vi "DataTreeCtrl loadedDoc.vi"(8 "error in (no error)":errorcluster, 10 "RootPath":path, 11 "DataTreeCtrl in":refnum<class "DataTreeCtrl.lvclass">) -> (0 "error out":errorcluster, 3 "DataTreeCtrl out":refnum<class "DataTreeCtrl.lvclass">)   [LabVIEW 2018, in "DataTreeCtrl.lvclass"]
uses:
  DataTreeCtrl.lvclass
  <vilib>/picture/picture.llb/imagedata.ctl
  DataTreeCtrl.lvclass/DataTreeCtrl.ctl
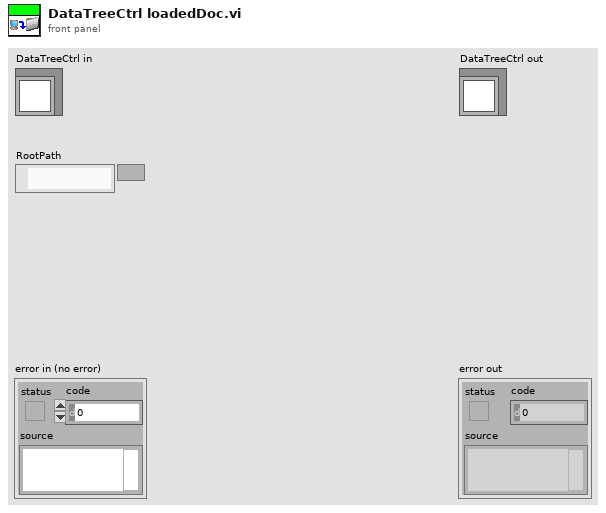
[diagram p1: front panel]
types:
  T1 = cluster{"Left Cell String":string, "Child Text":string[], "Child Tag":string, "Item Indent":i32, "Child Only?":bool, "Glyph Index":i32}
  T2 = typedef "imagedata.ctl" = cluster{"image type":i32, "image depth":i32, "image":u8[], "mask":u8[], "colors":u32[], "Rectangle":cluster{"left":i16, "top":i16, "right":i16, "bottom":i16}}
  T3 = cluster{"Left Cell String":string, "Child Text":string[], "Child Tag":string, "Item Indent":i32, "Child Only?":bool, "Glyph Index":i32}[]
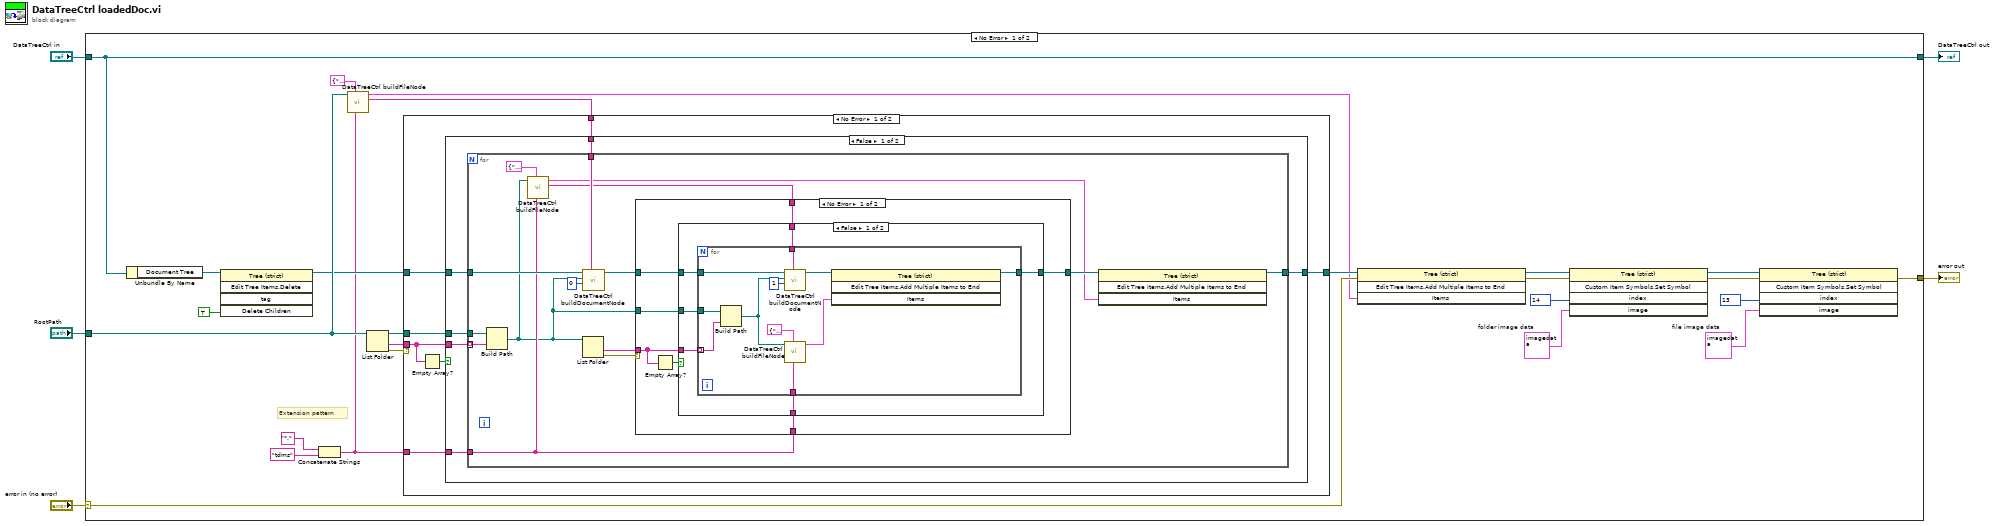
[diagram p0: block diagram]
diagram:
  n1 = case shown="No Error" "error in (no error)" {
    selector: "error in (no error)" -> [w19 w88]
    tunnel: [w17 w88] -> w1
    tunnel: [w10 w87] -> w4
    tunnel: "DataTreeCtrl in" -> [w10 w87]
    tunnel: "RootPath" -> [w13 _]
    frame No Error {
      w28 = T2 {"image type"=0, "image depth"=32, "image"=[0, 0, 0, 0, 0, 0, 0, 0, 0, 0, 0, 0, 0, 0, 0, 0, 0, 0, 0, 0, 0, 0, 0, 0, 0, 0, 0, 0, 0, 0, 0, 0, 0, 0, 0, 0, 0, 0, 0, 0, 0, 0, 0, 0, 0, 0, 0, 0, 0, 0, 0, 0, 0, 0, 0, 0, 0, 0, 0, 0, 0, 0, 0, 0, 0, 0, 0, 0, 0, 0, 0, 0, 0, 0, 0, 0, 0, 0, 0, 0, 0, 0, 0, 0, 0, 0, 0, 0, 0, 0, 0, 0, 0, 0, 0, 0, 0, 0, 0, 0, 0, 0, 0, 0, 0, 0, 0, 0, 0, 0, 0, 0, 0, 0, 0, 0, 0, 0, 0, 0, 0, 0, 0, 0, 0, 0, 0, 0, 0, 0, 0, 0, 0, 0, 0, 0, 0, 0, 0, 0, 0, 0, 0, 0, 0, 0, 0, 0, 0, 0, 0, 0, 0, 0, 0, 0, 0, 0, 0, 0, 0, 0, 0, 0, 0, 0, 0, 0, 0, 0, 0, 0, 0, 0, 0, 0, 0, 0, 0, 0, 0, 0, 0, 0, 0, 0, 0, 0, 0, 0, 0, 0, 0, 0, 0, 0, 0, 0, 0, 0, 0, 0, 0, 0, 0, 0, 0, 0, 0, 0, 0, 0, 0, 0, 0, 0, 0, 0, 0, 0, 0, 0, 0, 0, 0, 0, 0, 0, 0, 0, 0, 0, 0, 0, 0, 0, 255, 0, 141, 202, 0, 0, 0, 0, 0, 0, 0, 0, 0, 0, 0, 0, 0, 0, 0, 0, 0, 0, 0, 0, 0, 0, 0, 0, 0, 0, 0, 0, 0, 0, 0, 0, 0, 0, 0, 0, 0, 0, 0, 0, 0, 0, 0, 0, 0, 0, 0, 0, 0, 0, 0, 0, 0, 0, 0, 0, 0, 0, 0, 0, 255, 0, 141, 202, 0, 0, 0, 0, 0, 0, 0, 0, 0, 0, 0, 0, 0, 0, 0, 0, 0, 0, 0, 0, 0, 0, 0, 0, 0, 0, 0, 0, 0, 0, 0, 0, 0, 0, 0, 0, 0, 0, 0, 0, 0, 0, 0, 0, 0, 0, 0, 0, 0, 0, 0, 0, 0, 0, 0, 0, 0, 0, 0, 0, 255, 0, 141, 202, 0, 0, 0, 0, 0, 0, 0, 0, 0, 0, 0, 0, 0, 0, 0, 0, 0, 0, 0, 0, 0, 0, 0, 0, 0, 0, 0, 0, 0, 0, 0, 0, 0, 0, 0, 0, 0, 0, 0, 0, 0, 0, 0, 0, 0, 0, 0, 0, 0, 0, 0, 0, 0, 0, 0, 0, 0, 0, 0, 0, 255, 0, 141, 202, 0, 0, 0, 0, 0, 0, 0, 0, 0, 0, 0, 0, 0, 0, 0, 0, 0, 0, 0, 0, 0, 0, 0, 0, 0, 0, 0, 0, 0, 0, 0, 0, 0, 0, 0, 0, 0, 0, 0, 0, 0, 0, 0, 0, 255, 0, 141, 202, 0, 0, 0, 0, 0, 0, 0, 0, 0, 0, 0, 0, 255, 0, 141, 202, 0, 0, 0, 0, 0, 0, 0, 0, 0, 0, 0, 0, 255, 0, 141, 202, 0, 0, 0, 0, 0, 0, 0, 0, 0, 0, 0, 0, 0, 0, 0, 0, 0, 0, 0, 0, 0, 0, 0, 0, 0, 0, 0, 0, 255, 0, 141, 202, 0, 0, 0, 0, 0, 0, 0, 0, 0, 0, 0, 0, 255, 0, 141, 202, 0, 0, 0, 0, 255, 0, 141, 202, 0, 0, 0, 0, 255, 0, 141, 202, 0, 0, 0, 0, 0, 0, 0, 0, 0, 0, 0, 0, 0, 0, 0, 0, 0, 0, 0, 0, 0, 0, 0, 0, 0, 0, 0, 0, 255, 0, 141, 202, 0, 0, 0, 0, 0, 0, 0, 0, 0, 0, 0, 0, 255, 0, 141, 202, 0, 0, 0, 0, 255, 0, 141, 202, 0, 0, 0, 0, 255, 0, 141, 202, 0, 0, 0, 0, 0, 0, 0, 0, 0, 0, 0, 0, 255, 0, 141, 202, 0, 0, 0, 0, 0, 0, 0, 0, 0, 0, 0, 0, 255, 0, 141, 202, 0, 0, 0, 0, 0, 0, 0, 0, 0, 0, 0, 0, 255, 0, 141, 202, 0, 0, 0, 0, 255, 0, 141, 202, 0, 0, 0, 0, 255, 0, 141, 202, 0, 0, 0, 0, 255, 0, 141, 202, 0, 0, 0, 0, 255, 0, 141, 202, 0, 0, 0, 0, 0, 0, 0, 0, 0, 0, 0, 0, 255, 0, 141, 202, 0, 0, 0, 0, 255, 0, 141, 202, 0, 0, 0, 0, 255, 0, 141, 202, 0, 0, 0, 0, 255, 0, 141, 202, 0, 0, 0, 0, 255, 0, 141, 202, 0, 0, 0, 0, 255, 0, 141, 202, 0, 0, 0, 0, 255, 0, 141, 202, 0, 0, 0, 0, 255, 0, 141, 202, 0, 0, 0, 0, 255, 0, 141, 202, 0, 0, 0, 0, 255, 0, 141, 202, 0, 0, 0, 0, 255, 0, 141, 202, 0, 0, 0, 0, 255, 0, 141, 202, 0, 0, 0, 0, 255, 0, 141, 202, 0, 0, 0, 0, 255, 0, 141, 202, 0, 0, 0, 0, 255, 0, 141, 202, 0, 0, 0, 0, 255, 0, 141, 202, 0, 0, 0, 0, 255, 0, 141, 202, 0, 0, 0, 0, 255, 0, 141, 202, 0, 0, 0, 0, 255, 0, 141, 202, 0, 0, 0, 0, 255, 0, 141, 202, 0, 0, 0, 0, 255, 0, 141, 202, 255, 0, 0, 0, 255, 0, 0, 0, 255, 0, 0, 0, 255, 0, 0, 0, 255, 0, 0, 0, 255, 0, 0, 0, 255, 0, 0, 0, 255, 0, 0, 0, 255, 0, 0, 0, 255, 0, 0, 0, 255, 0, 0, 0, 255, 0, 0, 0, 255, 0, 0, 0, 255, 0, 0, 0, 255, 0, 0, 0, 255, 0, 0, 0, 0, 0, 0, 0, 0, 0, 0, 0, 0, 0, 0, 0, 0, 0, 0, 0, 0, 0, 0, 0, 0, 0, 0, 0, 0, 0, 0, 0, 0, 0, 0, 0, 0, 0, 0, 0, 0, 0, 0, 0, 0, 0, 0, 0, 0, 0, 0, 0, 0, 0, 0, 0, 0, 0, 0, 0, 0, 0, 0, 0, 0, 0, 0, 0], "mask"=[0, 0, 0, 0, 0, 0, 0, 16, 0, 16, 0, 16, 0, 16, 1, 17, 1, 21, 1, 21, 17, 21, 81, 85, 85, 85, 85, 85, 255, 255, 0, 0], "colors"=[], "Rectangle"={"left"=0, "top"=0, "right"=16, "bottom"=16}}  # file image data
      w27 = T2 {"image type"=0, "image depth"=32, "image"=[16, 0, 0, 0, 16, 0, 0, 0, 16, 0, 0, 0, 16, 0, 0, 0, 16, 0, 0, 0, 12, 0, 0, 0, 0, 0, 0, 0, 0, 0, 0, 0, 0, 0, 0, 0, 0, 0, 0, 0, 0, 0, 0, 0, 0, 0, 0, 0, 0, 0, 0, 0, 0, 0, 0, 0, 0, 0, 0, 0, 0, 0, 0, 0, 255, 0, 0, 0, 255, 0, 0, 0, 255, 0, 0, 0, 255, 0, 0, 0, 255, 0, 0, 0, 248, 0, 0, 0, 44, 0, 0, 0, 0, 0, 0, 0, 0, 0, 0, 0, 0, 0, 0, 0, 0, 0, 0, 0, 0, 0, 0, 0, 0, 0, 0, 0, 0, 0, 0, 0, 0, 0, 0, 0, 0, 0, 0, 0, 255, 0, 0, 0, 255, 0, 0, 0, 255, 0, 0, 0, 255, 0, 0, 0, 255, 0, 0, 0, 255, 0, 0, 0, 209, 0, 0, 0, 48, 0, 0, 0, 48, 0, 0, 0, 48, 0, 0, 0, 48, 0, 0, 0, 48, 0, 0, 0, 48, 0, 0, 0, 48, 0, 0, 0, 48, 0, 0, 0, 48, 0, 0, 0, 255, 0, 0, 0, 255, 0, 0, 0, 255, 0, 0, 0, 255, 0, 0, 0, 255, 0, 0, 0, 255, 0, 0, 0, 255, 0, 0, 0, 202, 0, 0, 0, 88, 0, 0, 0, 88, 0, 0, 0, 88, 0, 0, 0, 88, 0, 0, 0, 88, 0, 0, 0, 88, 0, 0, 0, 88, 0, 0, 0, 177, 0, 0, 0, 255, 0, 0, 0, 255, 0, 0, 0, 255, 0, 0, 0, 255, 0, 0, 0, 255, 0, 0, 0, 255, 0, 0, 0, 255, 0, 0, 0, 254, 0, 0, 0, 116, 0, 0, 0, 88, 0, 0, 0, 88, 0, 0, 0, 88, 0, 0, 0, 88, 0, 0, 0, 88, 0, 0, 0, 88, 0, 0, 0, 177, 0, 0, 0, 255, 0, 0, 0, 255, 0, 0, 0, 255, 0, 0, 0, 255, 0, 0, 0, 255, 0, 0, 0, 255, 0, 0, 0, 255, 0, 0, 0, 255, 0, 0, 0, 255, 0, 0, 0, 255, 0, 0, 0, 255, 0, 0, 0, 255, 0, 0, 0, 255, 0, 0, 0, 255, 0, 0, 0, 255, 0, 0, 0, 255, 0, 0, 0, 255, 0, 0, 0, 255, 0, 0, 0, 255, 0, 0, 0, 255, 0, 0, 0, 255, 0, 0, 0, 255, 0, 0, 0, 255, 0, 0, 0, 255, 0, 0, 0, 255, 0, 0, 0, 255, 0, 0, 0, 255, 0, 0, 0, 255, 0, 0, 0, 255, 0, 0, 0, 255, 0, 0, 0, 255, 0, 0, 0, 255, 0, 0, 0, 255, 0, 0, 0, 255, 0, 0, 0, 255, 0, 0, 0, 255, 0, 0, 0, 246, 0, 0, 0, 152, 0, 0, 0, 152, 0, 0, 0, 152, 0, 0, 0, 157, 0, 0, 0, 254, 0, 0, 0, 255, 0, 0, 0, 255, 0, 0, 0, 255, 0, 0, 0, 255, 0, 0, 0, 255, 0, 0, 0, 255, 0, 0, 0, 255, 0, 0, 0, 255, 0, 0, 0, 255, 0, 0, 0, 255, 0, 0, 0, 255, 0, 0, 0, 224, 0, 0, 0, 224, 0, 0, 0, 224, 0, 0, 0, 228, 0, 0, 0, 255, 0, 0, 0, 255, 0, 0, 0, 255, 0, 0, 0, 255, 0, 0, 0, 255, 0, 0, 0, 255, 0, 0, 0, 255, 0, 0, 0, 255, 0, 0, 0, 255, 0, 0, 0, 255, 0, 0, 0, 255, 0, 0, 0, 246, 0, 0, 0, 121, 0, 0, 0, 120, 0, 0, 0, 120, 0, 0, 0, 120, 0, 0, 0, 120, 0, 0, 0, 121, 0, 0, 0, 246, 0, 0, 0, 255, 0, 0, 0, 255, 0, 0, 0, 255, 0, 0, 0, 255, 0, 0, 0, 255, 0, 0, 0, 255, 0, 0, 0, 255, 0, 0, 0, 255, 0, 0, 0, 254, 0, 0, 0, 208, 0, 0, 0, 208, 0, 0, 0, 208, 0, 0, 0, 208, 0, 0, 0, 208, 0, 0, 0, 208, 0, 0, 0, 254, 0, 0, 0, 255, 0, 0, 0, 255, 0, 0, 0, 255, 0, 0, 0, 255, 0, 0, 0, 255, 0, 0, 0, 255, 0, 0, 0, 255, 0, 0, 0, 255, 0, 0, 0, 248, 0, 0, 0, 168, 0, 0, 0, 168, 0, 0, 0, 168, 0, 0, 0, 168, 0, 0, 0, 168, 0, 0, 0, 168, 0, 0, 0, 248, 0, 0, 0, 255, 0, 0, 0, 255, 0, 0, 0, 255, 0, 0, 0, 255, 0, 0, 0, 255, 0, 0, 0, 255, 0, 0, 0, 255, 0, 0, 0, 255, 0, 0, 0, 255, 0, 0, 0, 255, 0, 0, 0, 255, 0, 0, 0, 255, 0, 0, 0, 255, 0, 0, 0, 255, 0, 0, 0, 255, 0, 0, 0, 255, 0, 0, 0, 255, 0, 0, 0, 255, 0, 0, 0, 255, 0, 0, 0, 255, 0, 0, 0, 255, 0, 0, 0, 255, 0, 0, 0, 255, 0, 0, 0, 255, 0, 0, 0, 255, 0, 0, 0, 255, 0, 0, 0, 255, 0, 0, 0, 255, 0, 0, 0, 255, 0, 0, 0, 255, 0, 0, 0, 255, 0, 0, 0, 255, 0, 0, 0, 255, 0, 0, 0, 255, 0, 0, 0, 255, 0, 0, 0, 255, 0, 0, 0, 255, 0, 0, 0, 255, 0, 0, 0, 255, 0, 0, 0, 255, 0, 0, 0, 255, 0, 0, 0, 255, 0, 0, 0, 255, 0, 0, 0, 255, 0, 0, 0, 255, 0, 0, 0, 255, 0, 0, 0, 255, 0, 0, 0, 255, 0, 0, 0, 255, 0, 0, 0, 255, 0, 0, 0, 255, 0, 0, 0, 255, 0, 0, 0, 16, 0, 0, 0, 16, 0, 0, 0, 16, 0, 0, 0, 16, 0, 0, 0, 16, 0, 0, 0, 16, 0, 0, 0, 16, 0, 0, 0, 16, 0, 0, 0, 16, 0, 0, 0, 16, 0, 0, 0, 16, 0, 0, 0, 16, 0, 0, 0, 16, 0, 0, 0, 16, 0, 0, 0, 16, 0, 0, 0, 16, 0, 0, 0], "mask"=[0, 0, 252, 0, 254, 0, 255, 1, 255, 1, 255, 255, 255, 255, 255, 255, 255, 255, 248, 31, 255, 255, 255, 255, 255, 255, 255, 255, 255, 255, 0, 0], "colors"=[], "Rectangle"={"left"=0, "top"=0, "right"=16, "bottom"=16}}  # folder image data
      # "Extension pattern"
      n2 = Unbundle By Name(w10) -> ("Document Tree"=w12:refnum<vi>)
      n3 = invoke class="Tree (strict)" method="Edit Tree Items.Delete"(reference=w12, "Delete Children"=TRUE ("Delete Children?")) -> (reference out=w9:refnum<vi>)  [unwired: 3 in, 4 out]
      n4 = Concatenate Strings("*." ("string"), "tdms" ("string")) -> (w6:string)
      n5 = call "DataTreeCtrl buildFileNode.vi"("Extension pattern"=w6, "Item"=T1 {"Left Cell String"="", "Child Text"=[], "Child Tag"="", "Item Indent"=0, "Child Only?"=TRUE, "Glyph Index"=0}, "RootPath"=w13) -> ("FileName"=w14:string[], "TreeItems"=w15:T3)  [unwired: 7 in]
      n6 = List Folder(path=w13) -> (path out=w30:path, folder names=w21:string[], error out=w29:errorcluster)  [unwired: 3 in, 1 out]
      n7 = case shown="No Error" w29 {
        tunnel: [w37 w86] -> w20
        tunnel: w21 -> [w32 _]
        tunnel: w9 -> [w35 w86]
        tunnel: w30 -> [w33 _]
        tunnel: w6 -> [w34 _]
        tunnel: w14 -> [w31 _]
        frame No Error {
          n8 = Empty Array?(array=w32) -> (empty?=w36:bool)
          n9 = case shown="False" w36 {
            tunnel: w32 -> [w43 _]
            tunnel: [w42 w85] -> w37
            tunnel: w35 -> [w41 w85]
            tunnel: w33 -> [w40 _]
            tunnel: w34 -> [w39 _]
            tunnel: w31 -> [w38 _]
            frame False {
              n10 = for {
                tunnel: w41 -> [w54]
                tunnel: w43 -> [w52] mode=indexing
                tunnel: w40 -> [w58]
                tunnel: [w56] -> w42
                tunnel: w39 -> [w49]
                tunnel: w38 -> [w46]
                n11 = Build Path(base path=w58, name or relative path=w52) -> (appended path=w47:path)
                n12 = call "DataTreeCtrl buildFileNode.vi"("Extension pattern"=w49, "Item"=T1 {"Left Cell String"="", "Child Text"=[], "Child Tag"="", "Item Indent"=1, "Child Only?"=TRUE, "Glyph Index"=0}, "RootPath"=w47) -> ("FileName"=w45:string[], "TreeItems"=w44:T3)  [unwired: 7 in]
                n13 = List Folder(path=w47) -> (folder names=w55:string[], error out=w50:errorcluster)  [unwired: 3 in, 2 out]
                n14 = call "DataTreeCtrl buildDocumentNode.vi"("FileName"=w46, "Indent"=0, "Root path"=w47, "Tree Ref In"=w54) -> ("Tree Ref Out"=w51:refnum<vi>)  [unwired: 7 in]
                n15 = case shown="No Error" w50 {
                  tunnel: [w65 w84] -> w57
                  tunnel: w55 -> [w64 _]
                  tunnel: w47 -> [w62 _]
                  tunnel: w51 -> [w61 w84]
                  tunnel: w49 -> [w60 _]
                  tunnel: w45 -> [w59 _]
                  frame No Error {
                    n16 = Empty Array?(array=w64) -> (empty?=w63:bool)
                    n17 = case shown="False" w63 {
                      tunnel: w62 -> [w70 _]
                      tunnel: [w68 w83] -> w65
                      tunnel: w64 -> [w69 _]
                      tunnel: w61 -> [w71 w83]
                      tunnel: w60 -> [w67 _]
                      tunnel: w59 -> [w66 _]
                      frame False {
                        n18 = for {
                          tunnel: w69 -> [w78] mode=indexing
                          tunnel: w70 -> [w82]
                          tunnel: [w81] -> w68
                          tunnel: w71 -> [w80]
                          tunnel: w67 -> [w75]
                          tunnel: w66 -> [w72]
                          n19 = Build Path(base path=w82, name or relative path=w78) -> (appended path=w73:path)
                          n20 = call "DataTreeCtrl buildDocumentNode.vi"("FileName"=w72, "Indent"=1, "Root path"=w73, "Tree Ref In"=w80) -> ("Tree Ref Out"=w77:refnum<vi>)  [unwired: 7 in]
                          n21 = call "DataTreeCtrl buildFileNode.vi"("Extension pattern"=w75, "Item"=T1 {"Left Cell String"="", "Child Text"=[], "Child Tag"="", "Item Indent"=2, "Child Only?"=TRUE, "Glyph Index"=0}, "RootPath"=w73) -> ("TreeItems"=w74:T3)  [unwired: 7 in, 1 out]
                          n22 = invoke class="Tree (strict)" method="Edit Tree Items.Add Multiple Items to End"(reference=w77, "Items"=w74) -> (reference out=w81:refnum<vi>)  [unwired: 2 in, 3 out]
                        }
                      }
                      frame True {
                      }
                    }
                  }
                  frame Error {
                  }
                }
                n23 = invoke class="Tree (strict)" method="Edit Tree Items.Add Multiple Items to End"(reference=w57, "Items"=w44) -> (reference out=w56:refnum<vi>)  [unwired: 2 in, 3 out]
              }
            }
            frame True {
            }
          }
        }
        frame Error {
        }
      }
      n24 = invoke class="Tree (strict)" method="Edit Tree Items.Add Multiple Items to End"(reference=w20, error in=w19, "Items"=w15) -> (reference out=w22:refnum<vi>, error out=w18:errorcluster)  [unwired: 1 in, 2 out]
      n25 = invoke class="Tree (strict)" method="Custom Item Symbols.Set Symbol"(reference=w22, error in=w18, "index"=14, "image"=w27) -> (reference out=w24:refnum<vi>, error out=w25:errorcluster)  [unwired: 1 in, 3 out]
      n26 = invoke class="Tree (strict)" method="Custom Item Symbols.Set Symbol"(reference=w24, error in=w25, "index"=13, "image"=w28) -> (error out=w17:errorcluster)  [unwired: 1 in, 4 out]
    }
    frame Error {
    }
  }
  "error out" <- w1
  "DataTreeCtrl out" <- w4
